vi "写触点.vi"(7 "布尔":bool, 8 "error out":errorcluster, 9 "触点类型":string, 10 "写入起始地址":string, 11 "VISA resource name out":refnum<visa-resource-name>) -> (0 "error IO":errorcluster, 2 "通讯延时":u32, 3 "VISA resource name out 2":refnum<visa-resource-name>)   [LabVIEW 2018]
uses:
  <vilib>/Instr/_visa.llb/VISA Configure Serial Port (Instr).vi
panel:
  out "连接的字符串":string
  out "读取缓冲区":string
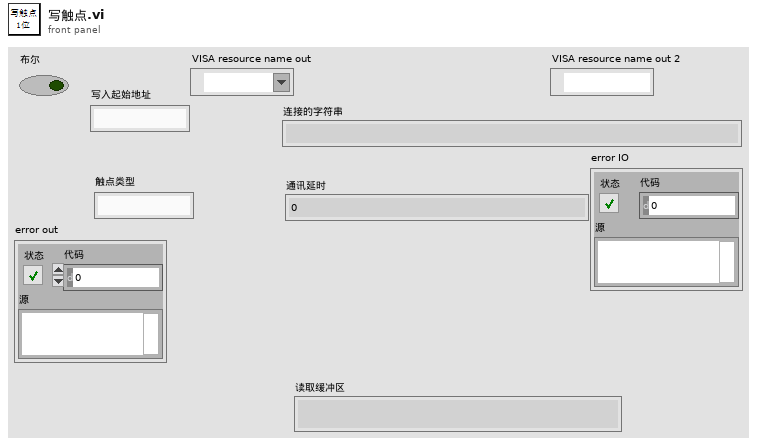
[diagram p1: front panel]
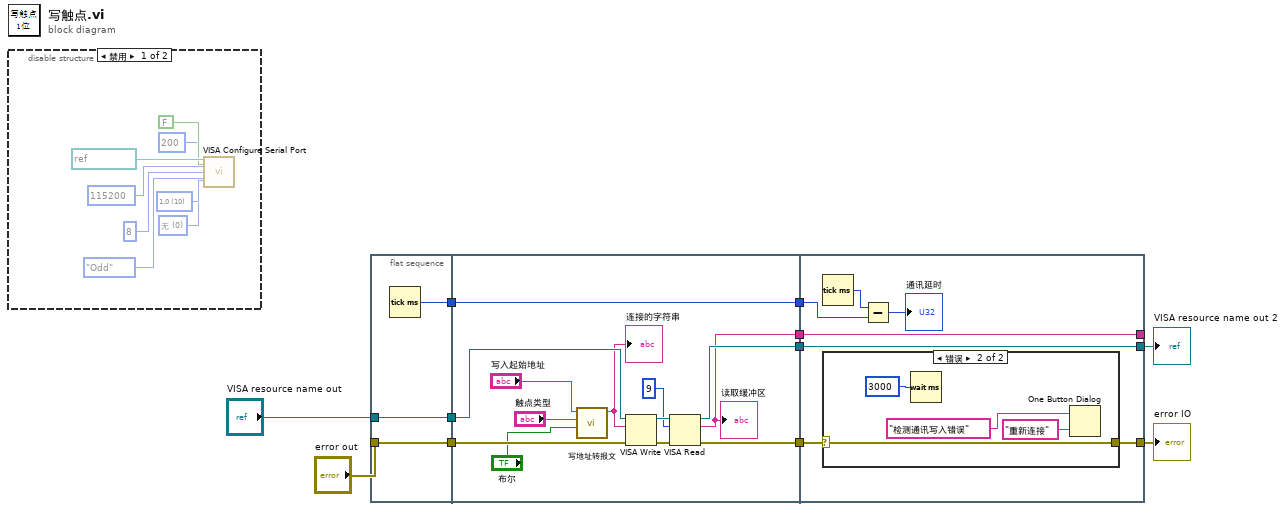
[diagram p0: block diagram]
diagram:
  n1 = disable-structure shown="禁用" {
    frame Disabled {
      w13 = u16 0 items=["无", "XON/XOFF", "RTS/CTS", "XON/XOFF & RTS/CTS", "DTR/DSR", "XON/XOFF & DTR/DSR"] ("flow control (0:none)")
      w14 = u16 10 items=["1.0"=10, "1.5"=15, "2.0"=20] ("stop bits (10: 1 bit)")
      n2 = call-poly "VISA Configure Serial Port"("VISA resource name"=refnum<visa-resource-name> "COM3", "timeout (10sec)"=u32 200, "Enable Termination\nChar (T)"=FALSE ("Enable Termination\nChar (T)"), "baud rate (9600)"=u32 115200, "data bits (8)"=u16 8, "parity (0:none)"=enum16{"None", "Odd", "Even", "Mark", "Space"}."Odd", "stop bits (10: 1 bit)"=w14, "flow control (0:none)"=w13) -> ()  [unwired: 6 in, 2 out]
    }
    frame Enabled {
    }
  }
  n3 = flat-sequence {
    tunnel: [w22] -> w11
    tunnel: "VISA resource name out" -> [w21]
    tunnel: [w21] -> w10
    tunnel: [w20] -> w9
    tunnel: "error out" -> [w20]
    tunnel: w11 -> [w35]
    tunnel: [w35] -> w8
    tunnel: [w34] -> w7
    tunnel: w10 -> [w33]
    tunnel: w9 -> [w32]
    tunnel: [w30] -> w6
    tunnel: [w26] -> w5
    tunnel: w8 -> [w41]
    tunnel: w7 -> [w39]
    tunnel: [w38] -> w1
    tunnel: w6 -> [w37]
    tunnel: [w37] -> w2
    tunnel: [w36] -> _
    tunnel: w5 -> [w36]
    frame #0 {
      n4 = Tick Count (ms)() -> (millisecond timer value=w22:u32)
    }
    frame #1 {
      n5 = call "写地址转报文.vi"("布尔"="布尔", "写入触点类型"="触点类型", "写入起始地址"="写入起始地址") -> ("连接的字符串"=w31:string)  [unwired: 8 in]
      "连接的字符串" <- w31
      n6 = VISA Write(VISA resource name=w33, write buffer=w31, error in (no error)=w32) -> (VISA resource name out=w29:refnum<visa-resource-name>, error out=w28:errorcluster)  [unwired: 1 out]
      n7 = VISA Read(VISA resource name=w29, byte count=u32 9 ("字节总数"), error in (no error)=w28) -> (VISA resource name out=w30:refnum<visa-resource-name>, read buffer=w26:string, error out=w34:errorcluster)  [unwired: 1 out]
      "读取缓冲区" <- w26
    }
    frame #2 {
      n8 = Tick Count (ms)() -> (millisecond timer value=w42:u32)
      n9 = case shown="错误" w39 {
        selector: w39 -> [w43 w47]
        tunnel: [w43 w47] -> w38
        frame No Error {
        }
        frame Error {
          n10 = Wait (ms)(milliseconds to wait=u32 3000 ("等待时间（毫秒）")) -> ()  [unwired: 1 out]
          n11 = One Button Dialog(message="检测通讯写入错误" ("消息"), button name ("OK")="重新连接" ("按钮名称（“确定”）")) -> ()  [unwired: 1 out]
        }
      }
      n12 = Subtract(x=w42, y=w41) -> (x-y=→"通讯延时":u32)
    }
  }
  "VISA resource name out 2" <- w2
  "error IO" <- w1
